vi "SVFA Peak Amplitude and Relative Phase (1x1).vi"(0 "reference signal X":waveform(dbl), 1 "response signal Y [EUy]":waveform(dbl), 2 "window":T9=1 items=["None"=0, "Hanning"=1, "Hamming"=2, "Blackman-Harris"=3, "Exact Blackman"=4, "Blackman"=5, "Flat Top"=6, "4 Term B-Harris "=7, "7 Term B-Harris"=8, "Low Sidelobe"=9, "Force - Exponential"=10, "Exponential"=65, "Blackman Nuttall"=11, "Triangle"=30, "Bartlett-Hanning"=31, "Bohman"=32, "Parzen"=33, "Welch"=34, "Kaiser"=60, "Dolph-Chebyshev"=61, "Gaussian"=62], 4 "view":T8={"dB On (T)"=FALSE, "unwrap phase (F)"=FALSE, "convert to degree (T)"=TRUE}, 5 "error in (no error)":errorcluster, 7 "averaging parameters":T7={"averaging mode"=enum."No averaging", "weighting mode"=enum."Exponential", "number of averages"=10, "linear mode"=enum."One shot"}, 8 "force and exponential window settings":cluster{"force [%]":dbl, "exponential [%]":dbl}={"force [%]"=50.0, "exponential [%]"=10.0} {"exponential [%]" min=0.0 max=100.0 format="%.2f"; "force [%]" min=0.0 max=100.0 format="%.2f"}, 9 "restart averaging (F)":bool) -> (11 "averaging done":bool, 12 "coherence":cluster{"f0":dbl, "df":dbl, "coherence":dbl[]} {"coherence" format="%.2f"; "df" format="%.2f"; "f0" format="%.2f"}, 13 "averages completed":dbl, 14 "magnitude [EUy pk]":cluster{"f0":dbl, "df":dbl, "magnitude":dbl[]} {"magnitude" format="%.2p"; "df" format="%.2p"; "f0" format="%.2p"}, 15 "magnitude unit label":string, 16 "phase":cluster{"f0":dbl, "df":dbl, "phase":dbl[]} {"phase" format="%.2f"; "df" format="%.2f"; "f0" format="%.2f"}, 17 "phase unit label":string, 18 "spectrum info":T1={"channel name"="", "description"="", "x-axis units"=0, "spectral info"={"spectrum type"=enum."Power [Magnitude^2]", "linear/dB"=enum."linear", "window"=0, "window size"=0, "FFT size"=0}, "engineering units"=0, "custom label"="", "dB reference [EU]"=0.0, "peak units"=enum."rms", "weighting filter"=0, "spectral density?"=FALSE, "unit label"="", "spectrum skewed?"=FALSE, "complimentary spectrum units"=enum."none"} {"x-axis units" items=["Time (s)"=0, "Frequency-CB (Hz)"=1, "Frequency-CPB (Hz)"=1248, "Frequency-Arbitrary (Hz)"=2357, "Quefrency (s)"=2, "Revolutions (rev)"=3, "Order"=4, "Speed (RPM)"=11, "Speed (rad/s)"=21, "Index"=65535]; "weighting filter" items=["Linear", "A-weighting", "B-weighting", "C-weighting", "ITU-R 468-4", "Dolby", "CCITT", "C-message", "Wb", "Wc", "Wd", "We", "Wf", "Wh", "Wj", "Wk", "Wm", "AES17 20 kHz lowpass", "AES17 40 kHz lowpass", "AES17 20 kHz highpass", "AES17 40 kHz highpass"]; "dB reference [EU]" format="%.2f"; "engineering units" items=["custom..."=0, "V"=1, "A"=21, "C"=30, "pC"=31, "s"=32, "-"=29, "Pa"=2, "N"=20, "g"=3, "m/s^2"=4, "m/s"=5, "m"=6, "mm/s"=12, "mm"=13, "micron/s"=14, "micron"=15, "in/s^2"=7, "in/s"=8, "in"=9, "mil/s"=10, "mil"=11, "rad/s^2"=16, "rad/s"=17, "rad"=18, "deg/s^2"=26, "deg/s"=27, "deg"=28, "RPM"=22, "cycle/s^2"=23, "Hz"=24, "cycle"=25, "strain"=19]; "spectral info"."window" items=["None "=0, "Hanning"=1, "Hamming"=2, "Blackman-Harris"=3, "Exact Blackman"=4, "Blackman"=5, "Flat Top"=6, "4 Term B-Harris "=7, "7 Term B-Harris"=8, "Low Sidelobe"=9, "Force - Exponential"=10, "Gaussian"=62]}, 19 "error out":errorcluster)   [LabVIEW 2017]
doc: "Use this VI to compute FFT spectra with magnitude equal to response magnitude and phase equal to response relative to reference. Use the N responses, 1 stimulus instance to compute phase-assigned auto spectra for multiple response channels."
uses:
  <vilib>/addons/_NISVFA/_Shared subVIs/Controls/svc_Window [Dual FFT].ctl
  <vilib>/addons/_NISVFA/_Shared subVIs/Controls/svc_Spectrum Info.ctl
  <vilib>/addons/_NISVFA/_Shared subVIs/Controls/svc_X-Axis Units.ctl
  <vilib>/addons/_NISVFA/_Shared subVIs/Controls/svc_Spectrum Type.ctl
  <vilib>/addons/_NISVFA/_Shared subVIs/Controls/svc_Engineering Units Text Ring.ctl
  <vilib>/addons/_NISVFA/_Shared subVIs/Controls/svc_Weighting Filter Text Ring.ctl
  <vilib>/addons/_NISVFA/_Shared subVIs/Controls/svc_Complimentary Spectrum Units.ctl
  <vilib>/addons/_NISVFA/_Shared subVIs/Controls/svc_Window.ctl
  <vilib>/addons/_NISVFA/_Spectrum Processing/SVFA Unit Conversion (1 Ch).vi
  <vilib>/addons/_NISVFA/_Shared subVIs/Windowing/svfa_Scaled Time Domain Window (1 Ch).vi
  <vilib>/addons/_NISVFA/_Shared subVIs/Common/svc_Spectrum Units.vi
  <vilib>/addons/_NISVFA/_Spectrum Processing/subVIs/svfa_Conversion Utility (spectrum info).vi
  <vilib>/addons/_NISVFA/_Shared subVIs/Windowing/svfa_Scaled Time Domain Window (Array).vi
  <vilib>/addons/_NISVFA/_Spectrum Processing/subVIs/svfa_Peak to RMS to Peak2Peak.vi
  <vilib>/addons/_NISVFA/_Spectrum Processing/subVIs/svfa_Mag to Mag2.vi
  <vilib>/addons/_NISVFA/_Spectrum Processing/subVIs/svfa_Linear to dB.vi
  <vilib>/addons/_NISVFA/_Spectrum Processing/subVIs/svfa_dBrefA to dBrefB.vi
  <vilib>/addons/_NISVFA/_Spectrum Processing/subVIs/svfa_Spectrum to Spectral Density.vi
  <vilib>/Analysis/4window.llb/Force Window.vi
  <vilib>/Analysis/4window.llb/Force Window (DBL).vi
  <vilib>/Analysis/4window.llb/Exponential Window.vi
  <vilib>/Analysis/4window.llb/Exponential Window (DBL).vi
  <vilib>/addons/_NISVFA/_Shared subVIs/Common/svc_Get Weighting Enum and Labels.vi
  <vilib>/addons/_NISVFA/_Shared subVIs/Common/svc_Unit Label Lexical Class.vi
  <vilib>/addons/_NISVFA/_Shared subVIs/Common/svc_Engineering Units to Unit Label.vi
  <vilib>/addons/_NISVFA/_Shared subVIs/Common/svc_Format Value (DBL).vi
  <vilib>/addons/_NISVFA/_Shared subVIs/Common/svc_Window Parameters.vi
  <vilib>/addons/_NISVFA/_Baseband FFT/SVFA FFT Spectrum (Mag-Phase) (1 Ch).vi
  <vilib>/addons/_NISVFA/_Baseband FFT/SVFA Frequency Response (1x1) (Mag-Phase).vi
  <vilib>/Utility/error.llb/Error Cluster From Error Code.vi
  <vilib>/Analysis/0measdsp.llb/Scaled Time Domain Window.vi
  <vilib>/Analysis/0measdsp.llb/Scaled Time Domain Window (DBL).vi
  <vilib>/addons/_NISVFA/_Spectrum Processing/subVIs/svfa_Spectrum Info Window to windowTd Type Def.vi
  <vilib>/addons/_NISVFA/_Shared subVIs/Common/svc_Get Window Info.vi
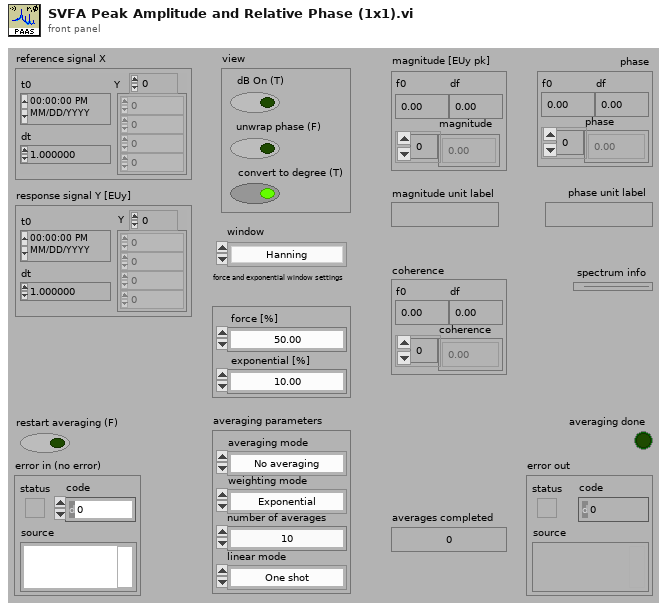
[diagram p1: front panel]
types:
  T1 = typedef "svc_Spectrum Info.ctl" = cluster{"channel name":string, "description":string, "x-axis units":T2, "spectral info":cluster{"spectrum type":T3, "linear/dB":enum16{"linear", "dB"}, "window":u16, "window size":i32, "FFT size":i32}, "engineering units":T4, "custom label":string, "dB reference [EU]":dbl, "peak units":enum16{"rms", "peak", "peak-peak"}, "weighting filter":T5, "spectral density?":bool, "unit label":string, "spectrum skewed?":bool, "complimentary spectrum units":T6}
  T2 = typedef "svc_X-Axis Units.ctl" = u16
  T3 = typedef "svc_Spectrum Type.ctl" = enum16{"FFT Spectrum [complex]", "Amplitude [Magnitude]", "Power [Magnitude^2]", "Cross Spectrum [complex]", "Frequency Response [Complex]"}
  T4 = typedef "svc_Engineering Units Text Ring.ctl" = u16
  T5 = typedef "svc_Weighting Filter Text Ring.ctl" = u16
  T6 = typedef "svc_Complimentary Spectrum Units.ctl" = enum16{"none", "radians", "degrees", "cycles", "imaginary"}
  T7 = cluster{"averaging mode":enum16{"No averaging", "Vector averaging", "RMS averaging", "Peak hold"}, "weighting mode":enum16{"Linear", "Exponential"}, "number of averages":u32, "linear mode":enum16{"One shot", "Auto restart"}}
  T8 = cluster{"dB On (T)":bool, "unwrap phase (F)":bool, "convert to degree (T)":bool}
  T9 = typedef "svc_Window [Dual FFT].ctl" = u32
  T10 = cluster{"linear/dB":enum16{"no change", "linear", "dB"}, "dB reference (0: no change)":dbl, "power/magnitude":enum16{"no change", "power", "magnitude"}, "view":enum16{"no change", "rms", "peak", "peak-peak"}}
  T11 = cluster{"dB On":bool, "unwrap phase":bool, "convert to degree":bool}
  T12 = typedef "svc_Window.ctl" = u32
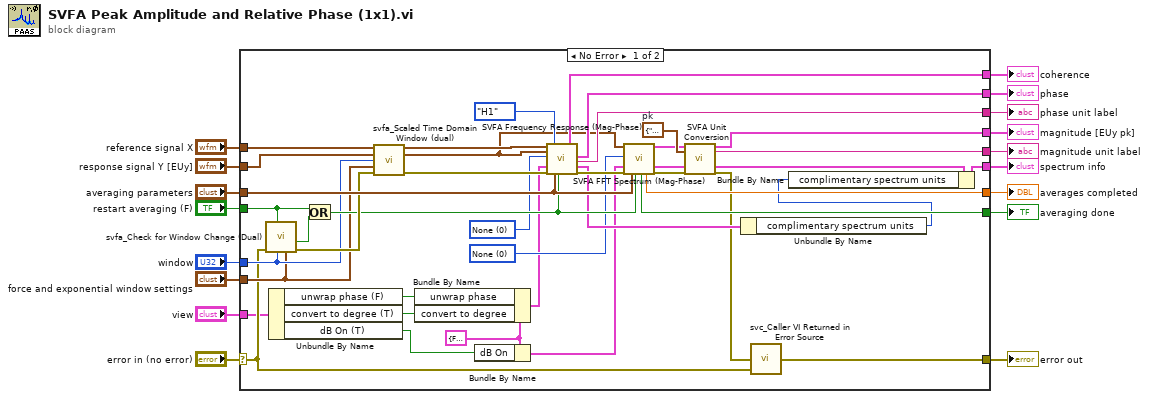
[diagram p0: block diagram]
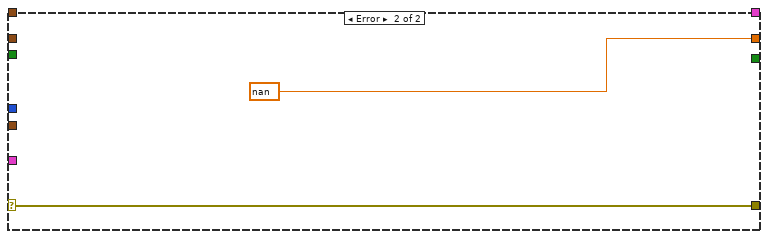
[diagram p2: hidden frame]
diagram:
  n1 = case shown="No Error" "error in (no error)" {
    selector: "error in (no error)" -> [w41 w60]
    tunnel: [w28 _] -> w17
    tunnel: [w57 _] -> w16
    tunnel: [w29 nan ("averages completed")] -> w15
    tunnel: [w56 _] -> w14
    tunnel: [w55 _] -> w13
    tunnel: [w27 _] -> w12
    tunnel: [w23 _] -> w11
    tunnel: [w22 _] -> w10
    tunnel: "view" -> [w36 _]
    tunnel: "averaging parameters" -> [w53 _]
    tunnel: "restart averaging (F)" -> [w50 _]
    tunnel: "window" -> [w48 _]
    tunnel: "force and exponential window settings" -> [w47 _]
    tunnel: "reference signal X" -> [w46 _]
    tunnel: "response signal Y [EUy]" -> [w44 _]
    tunnel: [w42 w60] -> w2
    frame No Error {
      w25 = T10 {"linear/dB"=enum."no change", "dB reference (0: no change)"=0.0, "power/magnitude"=enum."no change", "view"=enum."peak"}  # pk
      w38 = T11 {"dB On"=FALSE, "unwrap phase"=FALSE, "convert to degree"=FALSE} ("view")
      w39 = T12 0 items=["None"=0, "Hanning"=1, "Hamming"=2, "Blackman-Harris"=3, "Exact Blackman"=4, "Blackman"=5, "Flat Top"=6, "4 Term B-Harris "=7, "7 Term B-Harris"=8, "Low Sidelobe"=9, "Blackman Nuttall"=11, "Triangle"=30, "Bartlett-Hanning"=31, "Bohman"=32, "Parzen"=33, "Welch"=34, "Kaiser"=60, "Dolph-Chebyshev"=61, "Gaussian"=62] ("window")
      w31 = T9 0 items=["None"=0, "Hanning"=1, "Hamming"=2, "Blackman-Harris"=3, "Exact Blackman"=4, "Blackman"=5, "Flat Top"=6, "4 Term B-Harris "=7, "7 Term B-Harris"=8, "Low Sidelobe"=9, "Force - Exponential"=10, "Blackman Nuttall"=11, "Triangle"=30, "Bartlett-Hanning"=31, "Bohman"=32, "Parzen"=33, "Welch"=34, "Kaiser"=60, "Dolph-Chebyshev"=61, "Gaussian"=62] ("window")
      n2 = call <vilib>:"svfa_Check for Window Change (Dual).vi"("force/exp settings"=w47, "window"=w48, "restart averaging (F)"=w50, "error in (no error)"=w41) -> ("error out"=w52:errorcluster, "parameter has changed"=w51:bool)  [unwired: 6 in]
      n3 = Unbundle By Name(w36) -> ("unwrap phase (F)"=w34:bool, "convert to degree (T)"=w33:bool, "dB On (T)"=w32:bool)
      n4 = Or(x=w50, y=w51) -> (x .or. y?=w49:bool)
      n5 = call <vilib>:"svfa_Scaled Time Domain Window (dual).vi"("Signal in [X]"=w46, "Signal in [Y]"=w44, "window"=w48, "force/exp settings"=w47, "error in (no error)"=w52) -> ("Windowed signal [X]"=w45:waveform(dbl), "Windowed signal [Y]"=w30:waveform(dbl), "error out"=w43:errorcluster)  [unwired: 4 in, 4 out]
      n6 = Bundle By Name(cluster=w38, "unwrap phase"=w34, "convert to degree"=w33) -> (w37:T11)
      n7 = Bundle By Name(cluster=w38, "dB On"=w32) -> (w35:T11)
      n8 = call-poly <vilib>:"SVFA Frequency Response (Mag-Phase).vi"("stimulus signal X [EUx]"=w45, "response signal Y [EUy]"=w30, "window"=w31, "view"=w37, "error in (no error)"=w43, "FRF mode"=enum16{"H1", "H2", "H3"}."H1", "averaging parameters"=w53, "restart averaging (F)"=w49) -> ("coherence"=w57:cluster{"f0":dbl, "df":dbl, "coherence":dbl[]}, "phase [degrees]"=w56:cluster{"f0":dbl, "df":dbl, "phase":dbl[]}, "phase unit label"=w55:string, "spectrum info"=w40:T1, "error out"=w54:errorcluster)  [unwired: 3 in, 4 out]
      n9 = call-poly <vilib>:"SVFA FFT Spectrum (Mag-Phase).vi"("scaled signal [EU]"=w30, "window"=w39, "view"=w35, "error in (no error)"=w54, "averaging parameters"=w53, "restart averaging (F)"=w49) -> ("averaging done"=w28:bool, "averages completed"=w29:dbl, "magnitude [dB EU]"=w24:cluster{"f0":dbl, "df":dbl, "magnitude":dbl[]}, "spectrum info"=w21:T1, "error out"=w19:errorcluster)  [unwired: 6 in, 3 out]
      n10 = call-poly <vilib>:"SVFA Unit Conversion.vi"("spectrum"=w24, "desired scaling"=w25, "spectrum info in"=w21, "error in (no error)"=w19) -> ("converted spectrum"=w23:cluster{"x0":dbl, "dx":dbl, "magnitude":dbl[]}, "unit label"=w22:string, "spectrum info out"=w20:T1, "error out"=w18:errorcluster)  [unwired: 12 in]
      n11 = Unbundle By Name(w40) -> ("complimentary spectrum units"=w26:T6)
      n12 = call <vilib>:"svc_Caller VI Returned in Error Source.vi"("warning input to caller"=w41, "error in (no error)"=w18) -> ("error out"=w42:errorcluster)  [unwired: 3 in]
      n13 = Bundle By Name(cluster=w20, "complimentary spectrum units"=w26) -> (w27:T1)
    }
    frame Error {
    }
  }
  "averaging done" <- w17
  "coherence" <- w16
  "averages completed" <- w15
  "magnitude [EUy pk]" <- w11
  "magnitude unit label" <- w10
  "phase" <- w14
  "phase unit label" <- w13
  "spectrum info" <- w12
  "error out" <- w2
